vi "BDF-Read Header.vi"(0 "Path":path=path "D:/Data/XYZ DATA/XYZ999/XYZ999-EFR3k110-28.0.0.bdf", 11 "error in":errorcluster) -> (4 "path out":path, 6 "Header":T1, 15 "error out":errorcluster)   [LabVIEW 2020]
uses:
  BDF-Header.ctl
  <vilib>/regexp/Match Regular Expression.xnode
panel:
  out "size (in bytes)":i64
  out "refnum out":refnum<file>
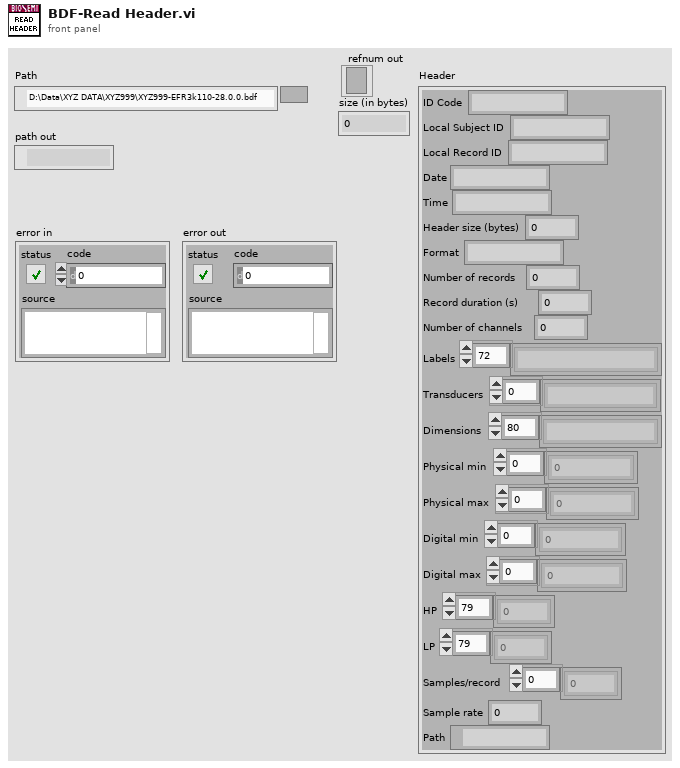
[diagram p1: front panel]
types:
  T1 = typedef "BDF-Header.ctl" = cluster{"ID Code":string, "Local Subject ID":string, "Local Record ID":string, "Date":string, "Time":string, "Header size (bytes)":i32, "Format":string, "Number of records":i32, "Record duration (s)":dbl, "Number of channels":i32, "Labels":string[], "Transducers":string[], "Dimensions":string[], "Physical min":dbl[], "Physical max":dbl[], "Digital min":i32[], "Digital max":i32[], "HP":dbl[], "LP":dbl[], "Samples/record":i32[], "Sample rate":dbl, "Path":path}
  T2 = enum16{"open", "replace", "create", "open or create", "replace or create", "replace or create with confirmation"}
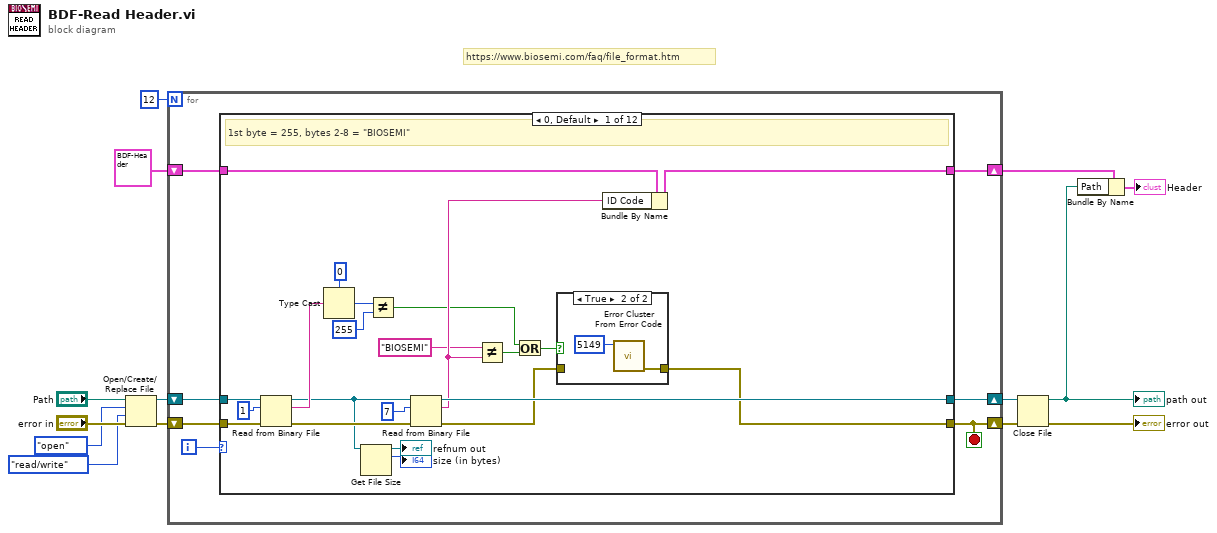
[diagram p0: block diagram]
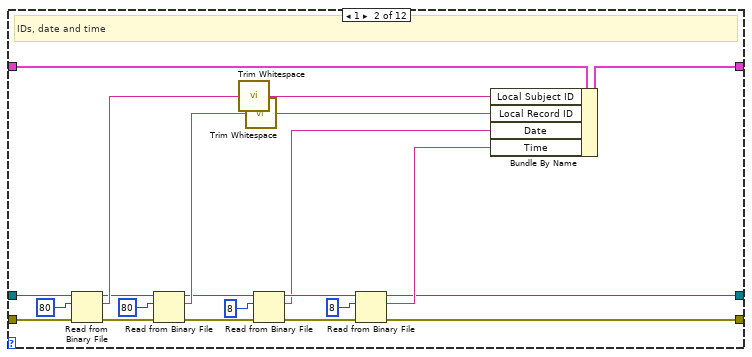
[diagram p3: hidden frame]
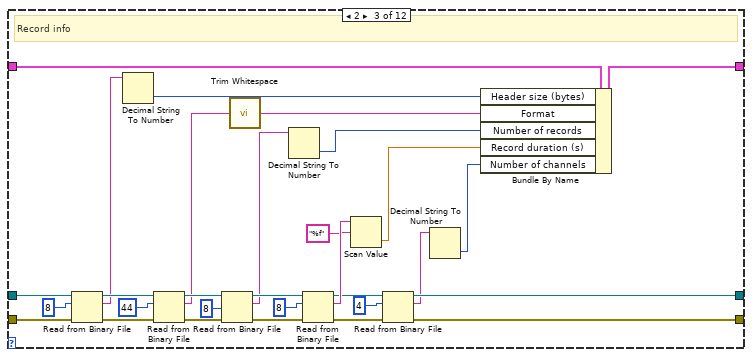
[diagram p4: hidden frame]
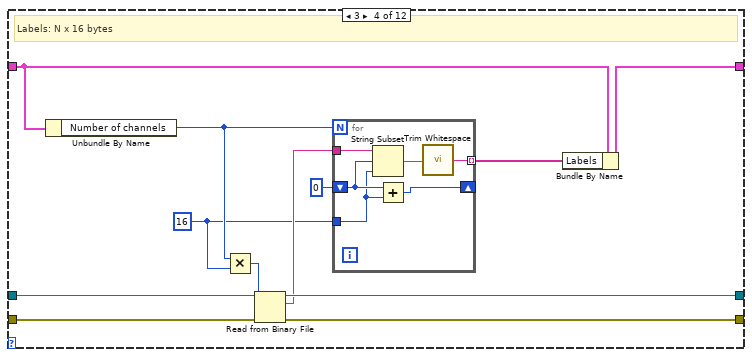
[diagram p5: hidden frame]
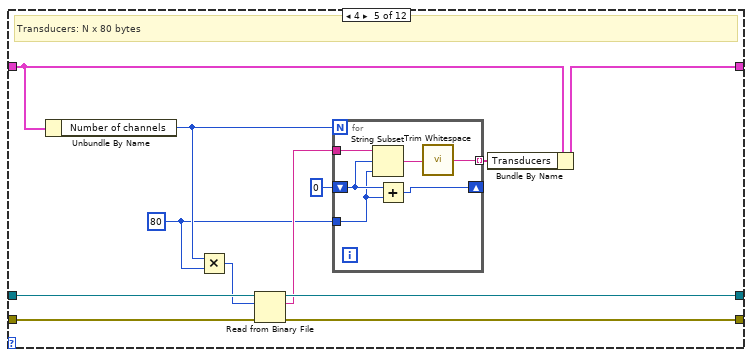
[diagram p6: hidden frame]
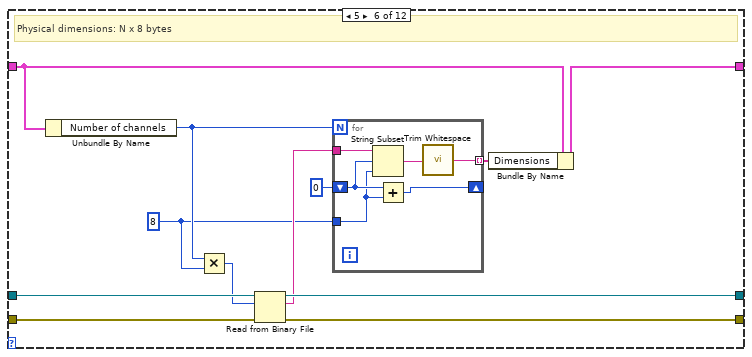
[diagram p7: hidden frame]
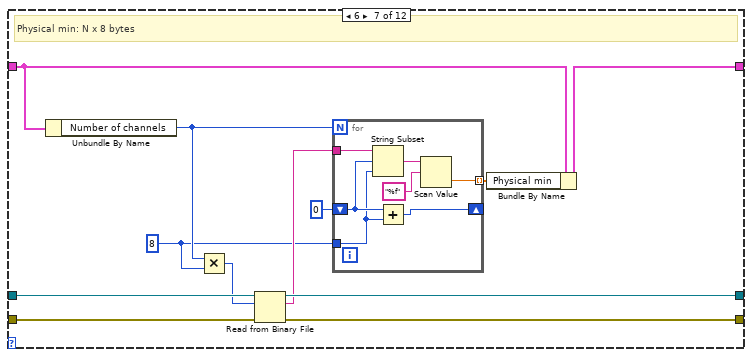
[diagram p8: hidden frame]
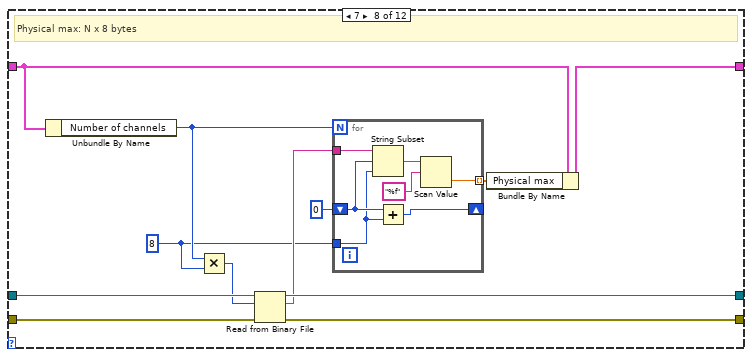
[diagram p9: hidden frame]
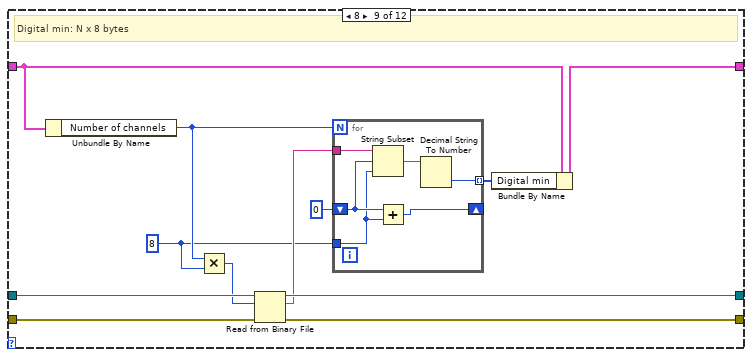
[diagram p10: hidden frame]
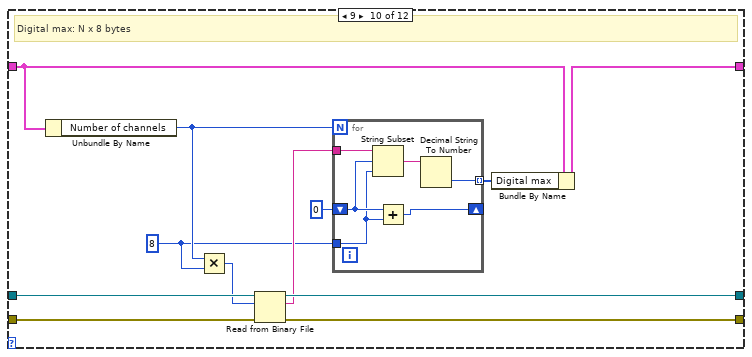
[diagram p11: hidden frame]
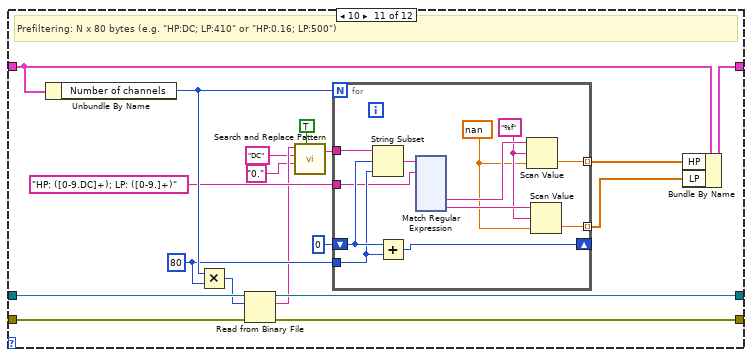
[diagram p12: hidden frame]
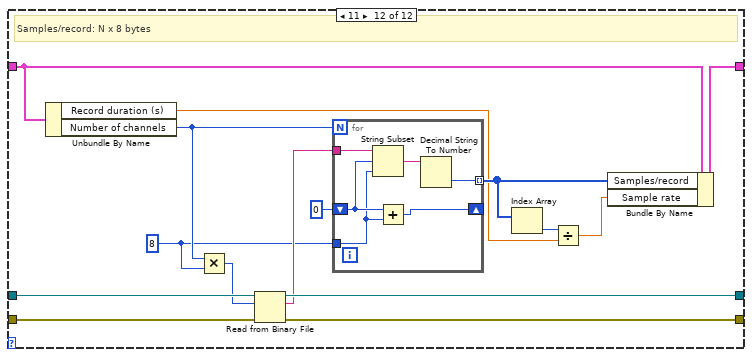
[diagram p13: hidden frame]
diagram:
  # "https://www.biosemi.com/faq/file_format.htm"
  n1 = Open/Create/Replace File(file path (use dialog)="Path", error in="error in", operation (0:open)=T2."open", access (0:read/write)=enum16{"read/write", "read-only", "write-only"}."read/write") -> (refnum out=w9:refnum<file>, error out=w10:errorcluster)  [unwired: 2 in, 1 out]
  n2 = for {
    N: 12 -> [_]
    shift-right: [w19] -> w8
    shift-left: w9 -> [w20]
    shift-right: [w15] -> w7
    shift-left: w10 -> [w21]
    shift-right: [w17] -> w6
    shift-left: T1 {"ID Code"="BIOSEMI", "Local Subject ID"="XYZ999", "Local Record ID"="EFR3k110-28.0", "Date"="12.08.19", "Time"="14.55.32", "Header size (bytes)"=20992, "Format"="24BIT", "Number of records"=18, "Record duration (s)"=1.0, "Number of channels"=81, "Labels"=["Fp1", "AF7", "AF3", "F1", "F3", "F5", "F7", "FT7", "FC5", "FC3", "FC1", "C1", "C3", "C5", "T7", "TP7", "CP5", "CP3", "CP1", "P1", "P3", "P5", "P7", "P9", "PO7", "PO3", "O1", "Iz", "Oz", "POz", "Pz", "CPz", "Fpz", "Fp2", "AF8", "AF4", "AFz", "Fz", "F2", "F4", "F6", "F8", "FT8", "FC6", "FC4", "FC2", "FCz", "Cz", "C2", "C4", "C6", "T8", "TP8", "CP6", "CP4", "CP2", "P2", "P4", "P6", "P8", "P10", "PO8", "PO4", "O2", "EXG1", "EXG2", "EXG3", "EXG4", "EXG5", "EXG6", "EXG7", "EXG8", "Status", "Status"], "Transducers"=["Active Electrode", "Active Electrode", "Active Electrode", "Active Electrode", "Active Electrode", "Active Electrode", "Active Electrode", "Active Electrode", "Active Electrode", "Active Electrode", "Active Electrode", "Active Electrode", "Active Electrode", "Active Electrode", "Active Electrode", "Active Electrode", "Active Electrode", "Active Electrode", "Active Electrode", "Active Electrode", "Active Electrode", "Active Electrode", "Active Electrode", "Active Electrode", "Active Electrode", "Active Electrode", "Active Electrode", "Active Electrode", "Active Electrode", "Active Electrode", "Active Electrode", "Active Electrode", "Active Electrode", "Active Electrode", "Active Electrode", "Active Electrode", "Active Electrode", "Active Electrode", "Active Electrode", "Active Electrode", "Active Electrode", "Active Electrode", "Active Electrode", "Active Electrode", "Active Electrode", "Active Electrode", "Active Electrode", "Active Electrode", "Active Electrode", "Active Electrode", "Active Electrode", "Active Electrode", "Active Electrode", "Active Electrode", "Active Electrode", "Active Electrode", "Active Electrode", "Active Electrode", "Active Electrode", "Active Electrode", "Active Electrode", "Active Electrode", "Active Electrode", "Active Electrode", "Active Electrode", "Active Electrode", "Active Electrode", "Active Electrode", "Active Electrode", "Active Electrode", "Active Electrode", "Active Electrode", "Analog Input Box", "Analog Input Box", "Analog Input Box", "Analog Input Box", "Analog Input Box", "Analog Input Box", "Analog Input Box", "Analog Input Box", "Triggers and Status"], "Dimensions"=["uV", "uV", "uV", "uV", "uV", "uV", "uV", "uV", "uV", "uV", "uV", "uV", "uV", "uV", "uV", "uV", "uV", "uV", "uV", "uV", "uV", "uV", "uV", "uV", "uV", "uV", "uV", "uV", "uV", "uV", "uV", "uV", "uV", "uV", "uV", "uV", "uV", "uV", "uV", "uV", "uV", "uV", "uV", "uV", "uV", "uV", "uV", "uV", "uV", "uV", "uV", "uV", "uV", "uV", "uV", "uV", "uV", "uV", "uV", "uV", "uV", "uV", "uV", "uV", "uV", "uV", "uV", "uV", "uV", "uV", "uV", "uV", "uV", "uV", "uV", "uV", "uV", "uV", "uV", "uV", "Boolean"], "Physical min"=[-262144.0, -262144.0, -262144.0, -262144.0, -262144.0, -262144.0, -262144.0, -262144.0, -262144.0, -262144.0, -262144.0, -262144.0, -262144.0, -262144.0, -262144.0, -262144.0, -262144.0, -262144.0, -262144.0, -262144.0, -262144.0, -262144.0, -262144.0, -262144.0, -262144.0, -262144.0, -262144.0, -262144.0, -262144.0, -262144.0, -262144.0, -262144.0, -262144.0, -262144.0, -262144.0, -262144.0, -262144.0, -262144.0, -262144.0, -262144.0, -262144.0, -262144.0, -262144.0, -262144.0, -262144.0, -262144.0, -262144.0, -262144.0, -262144.0, -262144.0, -262144.0, -262144.0, -262144.0, -262144.0, -262144.0, -262144.0, -262144.0, -262144.0, -262144.0, -262144.0, -262144.0, -262144.0, -262144.0, -262144.0, -262144.0, -262144.0, -262144.0, -262144.0, -262144.0, -262144.0, -262144.0, -262144.0, -1048576.0, -1048576.0, -1048576.0, -1048576.0, -1048576.0, -1048576.0, -1048576.0, -1048576.0, -8388608.0], "Physical max"=[262143.0, 262143.0, 262143.0, 262143.0, 262143.0, 262143.0, 262143.0, 262143.0, 262143.0, 262143.0, 262143.0, 262143.0, 262143.0, 262143.0, 262143.0, 262143.0, 262143.0, 262143.0, 262143.0, 262143.0, 262143.0, 262143.0, 262143.0, 262143.0, 262143.0, 262143.0, 262143.0, 262143.0, 262143.0, 262143.0, 262143.0, 262143.0, 262143.0, 262143.0, 262143.0, 262143.0, 262143.0, 262143.0, 262143.0, 262143.0, 262143.0, 262143.0, 262143.0, 262143.0, 262143.0, 262143.0, 262143.0, 262143.0, 262143.0, 262143.0, 262143.0, 262143.0, 262143.0, 262143.0, 262143.0, 262143.0, 262143.0, 262143.0, 262143.0, 262143.0, 262143.0, 262143.0, 262143.0, 262143.0, 262143.0, 262143.0, 262143.0, 262143.0, 262143.0, 262143.0, 262143.0, 262143.0, 1048575.0, 1048575.0, 1048575.0, 1048575.0, 1048575.0, 1048575.0, 1048575.0, 1048575.0, 8388607.0], "Digital min"=[-8388608, -8388608, -8388608, -8388608, -8388608, -8388608, -8388608, -8388608, -8388608, -8388608, -8388608, -8388608, -8388608, -8388608, -8388608, -8388608, -8388608, -8388608, -8388608, -8388608, -8388608, -8388608, -8388608, -8388608, -8388608, -8388608, -8388608, -8388608, -8388608, -8388608, -8388608, -8388608, -8388608, -8388608, -8388608, -8388608, -8388608, -8388608, -8388608, -8388608, -8388608, -8388608, -8388608, -8388608, -8388608, -8388608, -8388608, -8388608, -8388608, -8388608, -8388608, -8388608, -8388608, -8388608, -8388608, -8388608, -8388608, -8388608, -8388608, -8388608, -8388608, -8388608, -8388608, -8388608, -8388608, -8388608, -8388608, -8388608, -8388608, -8388608, -8388608, -8388608, -8388608, -8388608, -8388608, -8388608, -8388608, -8388608, -8388608, -8388608, -8388608], "Digital max"=[8388607, 8388607, 8388607, 8388607, 8388607, 8388607, 8388607, 8388607, 8388607, 8388607, 8388607, 8388607, 8388607, 8388607, 8388607, 8388607, 8388607, 8388607, 8388607, 8388607, 8388607, 8388607, 8388607, 8388607, 8388607, 8388607, 8388607, 8388607, 8388607, 8388607, 8388607, 8388607, 8388607, 8388607, 8388607, 8388607, 8388607, 8388607, 8388607, 8388607, 8388607, 8388607, 8388607, 8388607, 8388607, 8388607, 8388607, 8388607, 8388607, 8388607, 8388607, 8388607, 8388607, 8388607, 8388607, 8388607, 8388607, 8388607, 8388607, 8388607, 8388607, 8388607, 8388607, 8388607, 8388607, 8388607, 8388607, 8388607, 8388607, 8388607, 8388607, 8388607, 8388607, 8388607, 8388607, 8388607, 8388607, 8388607, 8388607, 8388607, 8388607], "HP"=[0.0, 0.0, 0.0, 0.0, 0.0, 0.0, 0.0, 0.0, 0.0, 0.0, 0.0, 0.0, 0.0, 0.0, 0.0, 0.0, 0.0, 0.0, 0.0, 0.0, 0.0, 0.0, 0.0, 0.0, 0.0, 0.0, 0.0, 0.0, 0.0, 0.0, 0.0, 0.0, 0.0, 0.0, 0.0, 0.0, 0.0, 0.0, 0.0, 0.0, 0.0, 0.0, 0.0, 0.0, 0.0, 0.0, 0.0, 0.0, 0.0, 0.0, 0.0, 0.0, 0.0, 0.0, 0.0, 0.0, 0.0, 0.0, 0.0, 0.0, 0.0, 0.0, 0.0, 0.0, 0.0, 0.0, 0.0, 0.0, 0.0, 0.0, 0.0, 0.0, 0.0, 0.0, 0.0, 0.0, 0.0, 0.0, 0.0, 0.0, nan], "LP"=[1667.0, 1667.0, 1667.0, 1667.0, 1667.0, 1667.0, 1667.0, 1667.0, 1667.0, 1667.0, 1667.0, 1667.0, 1667.0, 1667.0, 1667.0, 1667.0, 1667.0, 1667.0, 1667.0, 1667.0, 1667.0, 1667.0, 1667.0, 1667.0, 1667.0, 1667.0, 1667.0, 1667.0, 1667.0, 1667.0, 1667.0, 1667.0, 1667.0, 1667.0, 1667.0, 1667.0, 1667.0, 1667.0, 1667.0, 1667.0, 1667.0, 1667.0, 1667.0, 1667.0, 1667.0, 1667.0, 1667.0, 1667.0, 1667.0, 1667.0, 1667.0, 1667.0, 1667.0, 1667.0, 1667.0, 1667.0, 1667.0, 1667.0, 1667.0, 1667.0, 1667.0, 1667.0, 1667.0, 1667.0, 1667.0, 1667.0, 1667.0, 1667.0, 1667.0, 1667.0, 1667.0, 1667.0, 1667.0, 1667.0, 1667.0, 1667.0, 1667.0, 1667.0, 1667.0, 1667.0, nan], "Samples/record"=[8192, 8192, 8192, 8192, 8192, 8192, 8192, 8192, 8192, 8192, 8192, 8192, 8192, 8192, 8192, 8192, 8192, 8192, 8192, 8192, 8192, 8192, 8192, 8192, 8192, 8192, 8192, 8192, 8192, 8192, 8192, 8192, 8192, 8192, 8192, 8192, 8192, 8192, 8192, 8192, 8192, 8192, 8192, 8192, 8192, 8192, 8192, 8192, 8192, 8192, 8192, 8192, 8192, 8192, 8192, 8192, 8192, 8192, 8192, 8192, 8192, 8192, 8192, 8192, 8192, 8192, 8192, 8192, 8192, 8192, 8192, 8192, 8192, 8192, 8192, 8192, 8192, 8192, 8192, 8192, 8192], "Sample rate"=0.0, "Path"=path ""} ("Header") -> [w18]
    i -> [w16]
    stop <- w15 stop-if-true
    n3 = case shown="0, Default" w16 {
      tunnel: w21 -> [w43 w68 w98 w108 w126 w144 w162 w181 w200 w218 w242 w386]
      tunnel: w20 -> [w42 w67 w97 w109 w127 w145 w163 w182 w201 w219 w243 w387]
      tunnel: [w32 w50 w71 w106 w124 w142 w160 w179 w198 w216 w240 w384] -> w19
      tunnel: w18 -> [w38 w66 w96 w110 w128 w146 w164 w183 w202 w220 w244 w388]
      tunnel: [w34 w64 w94 w102 w118 w136 w154 w173 w192 w210 w235 w378] -> w17
      tunnel: [w25 w49 w72 w107 w125 w143 w161 w180 w199 w217 w241 w385] -> w15
      frame 0, Default {
        # "1st byte = 255, bytes 2-8 = \"BIOSEMI\""
        n4 = Read from Binary File(8:w43, 10:1 ("count (1)"), 11:w42) -> (0:w33:errorcluster, 2:w40:string, 3:w24:refnum<file>)  [unwired: 3 in, 1 out]
        n5 = Type Cast(type=u8 0, x=w40) -> (*(type *) &x=w37:u8)
        n6 = Get File Size(file=w24) -> (refnum out=→"refnum out":refnum<file>, size (in bytes)=→"size (in bytes)":i64)  [unwired: 1 in, 1 out]
        n7 = Not Equal?(x=w37, y=u8 255) -> (x != y?=w28:bool)
        n8 = Read from Binary File(8:w33, 10:7 ("count (1)"), 11:w24) -> (0:w26:errorcluster, 2:w31:string, 3:w32:refnum<file>)  [unwired: 3 in, 1 out]
        n9 = Not Equal?(x="BIOSEMI", y=w31) -> (x != y?=w29:bool)
        n10 = Or(x=w28, y=w29) -> (x .or. y?=w27:bool)
        n11 = case shown="True" w27 {
          tunnel: w26 -> [w44 _]
          tunnel: [w44 w46] -> w25
          frame False {
          }
          frame True {
            n12 = call <vilib>:"Error Cluster From Error Code.vi"("error code (0)"=5149) -> ("error out"=w46:errorcluster)  [unwired: 8 in]
          }
        }
        n13 = Bundle By Name(cluster=w38, "ID Code"=w31) -> (w34:T1)
      }
      frame 1 {
        # "IDs, date and time"
        n14 = Read from Binary File(8:w68, 10:80 ("count (1)"), 11:w67) -> (0:w60:errorcluster, 2:w63:string, 3:w61:refnum<file>)  [unwired: 3 in, 1 out]
        n15 = Read from Binary File(8:w60, 10:80 ("count (1)"), 11:w61) -> (0:w55:errorcluster, 2:w59:string, 3:w56:refnum<file>)  [unwired: 3 in, 1 out]
        n16 = call <vilib>:"Trim Whitespace.vi"("string"=w63) -> ("trimmed string"=w48:string)  [unwired: 1 in]
        n17 = call <vilib>:"Trim Whitespace.vi"("string"=w59) -> ("trimmed string"=w47:string)  [unwired: 1 in]
        n18 = Read from Binary File(8:w55, 10:8 ("count (1)"), 11:w56) -> (0:w53:errorcluster, 2:w52:string, 3:w54:refnum<file>)  [unwired: 3 in, 1 out]
        n19 = Read from Binary File(8:w53, 10:8 ("count (1)"), 11:w54) -> (0:w49:errorcluster, 2:w51:string, 3:w50:refnum<file>)  [unwired: 3 in, 1 out]
        n20 = Bundle By Name(cluster=w66, "Local Subject ID"=w48, "Local Record ID"=w47, "Date"=w52, "Time"=w51) -> (w64:T1)
      }
      frame 2 {
        # "Record info"
        n21 = Read from Binary File(8:w98, 10:8 ("count (1)"), 11:w97) -> (0:w91:errorcluster, 2:w84:string, 3:w92:refnum<file>)  [unwired: 3 in, 1 out]
        n22 = Decimal String To Number(string=w84) -> (number=w83:i32)  [unwired: 2 in, 1 out]
        n23 = Read from Binary File(8:w91, 10:44 ("count (1)"), 11:w92) -> (0:w87:errorcluster, 2:w82:string, 3:w88:refnum<file>)  [unwired: 3 in, 1 out]
        n24 = Read from Binary File(8:w87, 10:8 ("count (1)"), 11:w88) -> (0:w85:errorcluster, 2:w81:string, 3:w86:refnum<file>)  [unwired: 3 in, 1 out]
        n25 = call <vilib>:"Trim Whitespace.vi"("string"=w82) -> ("trimmed string"=w76:string)  [unwired: 1 in]
        n26 = Decimal String To Number(string=w81) -> (number=w80:i32)  [unwired: 2 in, 1 out]
        n27 = Read from Binary File(8:w85, 10:8 ("count (1)"), 11:w86) -> (0:w74:errorcluster, 2:w79:string, 3:w73:refnum<file>)  [unwired: 3 in, 1 out]
        n28 = Scan Value(string=w79, format string="%f") -> (value=w78:dbl)  [unwired: 1 in, 1 out]
        n29 = Read from Binary File(8:w74, 10:4 ("count (1)"), 11:w73) -> (0:w72:errorcluster, 2:w70:string, 3:w71:refnum<file>)  [unwired: 3 in, 1 out]
        n30 = Decimal String To Number(string=w70) -> (number=w69:i32)  [unwired: 2 in, 1 out]
        n31 = Bundle By Name(cluster=w96, "Header size (bytes)"=w83, "Format"=w76, "Number of records"=w80, "Record duration (s)"=w78, "Number of channels"=w69) -> (w94:T1)
      }
      frame 3 {
        w99 = 16
        # "Labels: N x 16 bytes"
        n32 = Unbundle By Name(w110) -> ("Number of channels"=w100:i32)
        n33 = Multiply(x=w100, y=w99) -> (x*y=w105:i32)
        n34 = Read from Binary File(8:w108, 10:w105, 11:w109) -> (0:w107:errorcluster, 2:w104:string, 3:w106:refnum<file>)  [unwired: 3 in, 1 out]
        n35 = for {
          N: w100 -> [_]
          tunnel: w104 -> [w116]
          tunnel: w99 -> [w114]
          shift-right: [w113] -> _
          shift-left: 0 -> [w115]
          tunnel: [w111] -> w101 mode=indexing
          n36 = String Subset(string=w116, offset (0)=w115, length (rest)=w114) -> (substring=w112:string)
          n37 = Add(x=w115, y=w114) -> (x+y=w113:i32)
          n38 = call <vilib>:"Trim Whitespace.vi"("string"=w112) -> ("trimmed string"=w111:string)  [unwired: 1 in]
        }
        n39 = Bundle By Name(cluster=w110, "Labels"=w101) -> (w102:T1)
      }
      frame 4 {
        w119 = 80
        # "Transducers: N x 80 bytes"
        n40 = Unbundle By Name(w128) -> ("Number of channels"=w122:i32)
        n41 = Multiply(x=w122, y=w119) -> (x*y=w123:i32)
        n42 = Read from Binary File(8:w126, 10:w123, 11:w127) -> (0:w125:errorcluster, 2:w121:string, 3:w124:refnum<file>)  [unwired: 3 in, 1 out]
        n43 = for {
          N: w122 -> [_]
          tunnel: w121 -> [w134]
          tunnel: w119 -> [w132]
          shift-right: [w131] -> _
          shift-left: 0 -> [w133]
          tunnel: [w129] -> w117 mode=indexing
          n44 = String Subset(string=w134, offset (0)=w133, length (rest)=w132) -> (substring=w130:string)
          n45 = Add(x=w133, y=w132) -> (x+y=w131:i32)
          n46 = call <vilib>:"Trim Whitespace.vi"("string"=w130) -> ("trimmed string"=w129:string)  [unwired: 1 in]
        }
        n47 = Bundle By Name(cluster=w128, "Transducers"=w117) -> (w118:T1)
      }
      frame 5 {
        w137 = 8
        # "Physical dimensions: N x 8 bytes"
        n48 = Unbundle By Name(w146) -> ("Number of channels"=w140:i32)
        n49 = Multiply(x=w140, y=w137) -> (x*y=w141:i32)
        n50 = Read from Binary File(8:w144, 10:w141, 11:w145) -> (0:w143:errorcluster, 2:w139:string, 3:w142:refnum<file>)  [unwired: 3 in, 1 out]
        n51 = for {
          N: w140 -> [_]
          tunnel: w139 -> [w152]
          tunnel: w137 -> [w150]
          shift-right: [w149] -> _
          shift-left: 0 -> [w151]
          tunnel: [w147] -> w135 mode=indexing
          n52 = String Subset(string=w152, offset (0)=w151, length (rest)=w150) -> (substring=w148:string)
          n53 = Add(x=w151, y=w150) -> (x+y=w149:i32)
          n54 = call <vilib>:"Trim Whitespace.vi"("string"=w148) -> ("trimmed string"=w147:string)  [unwired: 1 in]
        }
        n55 = Bundle By Name(cluster=w146, "Dimensions"=w135) -> (w136:T1)
      }
      frame 6 {
        w155 = 8
        # "Physical min: N x 8 bytes"
        n56 = Unbundle By Name(w164) -> ("Number of channels"=w158:i32)
        n57 = Multiply(x=w158, y=w155) -> (x*y=w159:i32)
        n58 = Read from Binary File(8:w162, 10:w159, 11:w163) -> (0:w161:errorcluster, 2:w157:string, 3:w160:refnum<file>)  [unwired: 3 in, 1 out]
        n59 = for {
          N: w158 -> [_]
          tunnel: w157 -> [w171]
          tunnel: w155 -> [w169]
          shift-right: [w168] -> _
          shift-left: 0 -> [w170]
          tunnel: [w165] -> w153 mode=indexing
          n60 = String Subset(string=w171, offset (0)=w170, length (rest)=w169) -> (substring=w167:string)
          n61 = Add(x=w170, y=w169) -> (x+y=w168:i32)
          n62 = Scan Value(string=w167, format string="%f") -> (value=w165:dbl)  [unwired: 1 in, 1 out]
        }
        n63 = Bundle By Name(cluster=w164, "Physical min"=w153) -> (w154:T1)
      }
      frame 7 {
        w174 = 8
        # "Physical max: N x 8 bytes"
        n64 = Unbundle By Name(w183) -> ("Number of channels"=w177:i32)
        n65 = Multiply(x=w177, y=w174) -> (x*y=w178:i32)
        n66 = Read from Binary File(8:w181, 10:w178, 11:w182) -> (0:w180:errorcluster, 2:w176:string, 3:w179:refnum<file>)  [unwired: 3 in, 1 out]
        n67 = for {
          N: w177 -> [_]
          tunnel: w176 -> [w190]
          tunnel: w174 -> [w188]
          shift-right: [w187] -> _
          shift-left: 0 -> [w189]
          tunnel: [w184] -> w172 mode=indexing
          n68 = String Subset(string=w190, offset (0)=w189, length (rest)=w188) -> (substring=w186:string)
          n69 = Add(x=w189, y=w188) -> (x+y=w187:i32)
          n70 = Scan Value(string=w186, format string="%f") -> (value=w184:dbl)  [unwired: 1 in, 1 out]
        }
        n71 = Bundle By Name(cluster=w183, "Physical max"=w172) -> (w173:T1)
      }
      frame 8 {
        w193 = 8
        # "Digital min: N x 8 bytes"
        n72 = Unbundle By Name(w202) -> ("Number of channels"=w196:i32)
        n73 = Multiply(x=w196, y=w193) -> (x*y=w197:i32)
        n74 = Read from Binary File(8:w200, 10:w197, 11:w201) -> (0:w199:errorcluster, 2:w195:string, 3:w198:refnum<file>)  [unwired: 3 in, 1 out]
        n75 = for {
          N: w196 -> [_]
          tunnel: w195 -> [w208]
          tunnel: w193 -> [w206]
          shift-right: [w205] -> _
          shift-left: 0 -> [w207]
          tunnel: [w203] -> w191 mode=indexing
          n76 = String Subset(string=w208, offset (0)=w207, length (rest)=w206) -> (substring=w204:string)
          n77 = Add(x=w207, y=w206) -> (x+y=w205:i32)
          n78 = Decimal String To Number(string=w204) -> (number=w203:i32)  [unwired: 2 in, 1 out]
        }
        n79 = Bundle By Name(cluster=w202, "Digital min"=w191) -> (w192:T1)
      }
      frame 9 {
        w211 = 8
        # "Digital max: N x 8 bytes"
        n80 = Unbundle By Name(w220) -> ("Number of channels"=w214:i32)
        n81 = Multiply(x=w214, y=w211) -> (x*y=w215:i32)
        n82 = Read from Binary File(8:w218, 10:w215, 11:w219) -> (0:w217:errorcluster, 2:w213:string, 3:w216:refnum<file>)  [unwired: 3 in, 1 out]
        n83 = for {
          N: w214 -> [_]
          tunnel: w213 -> [w226]
          tunnel: w211 -> [w224]
          shift-right: [w223] -> _
          shift-left: 0 -> [w225]
          tunnel: [w221] -> w209 mode=indexing
          n84 = String Subset(string=w226, offset (0)=w225, length (rest)=w224) -> (substring=w222:string)
          n85 = Add(x=w225, y=w224) -> (x+y=w223:i32)
          n86 = Decimal String To Number(string=w222) -> (number=w221:i32)  [unwired: 2 in, 1 out]
        }
        n87 = Bundle By Name(cluster=w220, "Digital max"=w209) -> (w210:T1)
      }
      frame 10 {
        w236 = 80
        # "Prefiltering: N x 80 bytes (e.g. \"HP:DC; LP:410\" or \"HP:0.16; LP:500\")"
        n88 = Unbundle By Name(w244) -> ("Number of channels"=w238:i32)
        n89 = Multiply(x=w238, y=w236) -> (x*y=w239:i32)
        n90 = Read from Binary File(8:w242, 10:w239, 11:w243) -> (0:w241:errorcluster, 2:w230:string, 3:w240:refnum<file>)  [unwired: 3 in, 1 out]
        n91 = call <vilib>:"Search and Replace Pattern.vi"("string"=w230, "regular expression (\"\")"="DC" ("regular expression (\"\")"), "replace string (\"\")"="0." ("replace string (\"\")"), "replace all? (F)"=TRUE) -> ("result string"=w231:string)  [unwired: 1 in, 1 out]
        n92 = for {
          N: w238 -> [_]
          tunnel: w231 -> [w256]
          tunnel: w236 -> [w254]
          shift-right: [w253] -> _
          shift-left: 0 -> [w255]
          tunnel: "HP: ([0-9.DC]+); LP: ([0-9.]+)" ("regular expression") -> [w252]
          tunnel: [w250] -> w233 mode=indexing
          tunnel: [w246] -> w232 mode=indexing
          w247 = nan
          w248 = "%f" ("format string")
          n93 = String Subset(string=w256, offset (0)=w255, length (rest)=w254) -> (substring=w245:string)
          n94 = Add(x=w255, y=w254) -> (x+y=w253:i32)
          n95 = xnode "Match Regular Expression"("input string"=w245, "regular expression"=w252) -> ("submatch 1"=w251:string, "submatch 2"=w249:string)  [unwired: 4 in, 5 out]
          n96 = Scan Value(string=w251, format string=w248, default (0 dbl)=w247) -> (value=w250:dbl)  [unwired: 1 out]
          n97 = Scan Value(string=w249, format string=w248, default (0 dbl)=w247) -> (value=w246:dbl)  [unwired: 1 out]
        }
        n98 = Bundle By Name(cluster=w244, "HP"=w233, "LP"=w232) -> (w235:T1)
      }
      frame 11 {
        w379 = 8
        # "Samples/record: N x 8 bytes"
        n99 = Unbundle By Name(w388) -> ("Record duration (s)"=w375:dbl, "Number of channels"=w382:i32)
        n100 = Multiply(x=w382, y=w379) -> (x*y=w383:i32)
        n101 = Read from Binary File(8:w386, 10:w383, 11:w387) -> (0:w385:errorcluster, 2:w381:string, 3:w384:refnum<file>)  [unwired: 3 in, 1 out]
        n102 = for {
          N: w382 -> [_]
          tunnel: w381 -> [w394]
          tunnel: w379 -> [w392]
          shift-right: [w391] -> _
          shift-left: 0 -> [w393]
          tunnel: [w389] -> w377 mode=indexing
          n103 = String Subset(string=w394, offset (0)=w393, length (rest)=w392) -> (substring=w390:string)
          n104 = Add(x=w393, y=w392) -> (x+y=w391:i32)
          n105 = Decimal String To Number(string=w390) -> (number=w389:i32)  [unwired: 2 in, 1 out]
        }
        n106 = Index Array(array=w377) -> (element=w376:i32)  [unwired: 1 in]
        n107 = Divide(x=w376, y=w375) -> (x/y=w374:dbl)
        n108 = Bundle By Name(cluster=w388, "Samples/record"=w377, "Sample rate"=w374) -> (w378:T1)
      }
    }
  }
  n109 = Close File(refnum=w8, error in=w7) -> (path=w1:path, error out=→"error out":errorcluster)
  "path out" <- w1
  n110 = Bundle By Name(cluster=w6, "Path"=w1) -> (→"Header":T1)
